vi "Item.vi"(8 "error in (no error)":errorcluster, 10 "Index":i32, 11 "ListImp in":refnum<class "ListImp.lvclass">) -> (0 "error out":errorcluster, 1 "Item":refnum<class>, 3 "ListImp out":refnum<class "ListImp.lvclass">)   [LabVIEW 2017, in "LapDog.Collections.v0.Lists.lvlib" / "ListImp.lvclass"]
uses:
  ListImp.lvclass
  ListImp.lvclass/ListImp.ctl
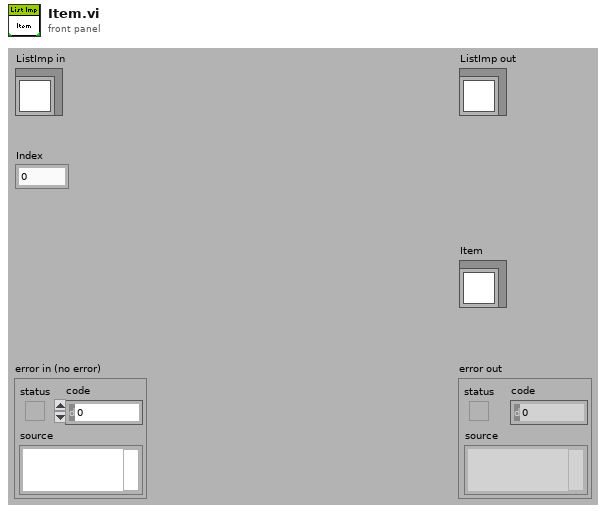
[diagram p1: front panel]
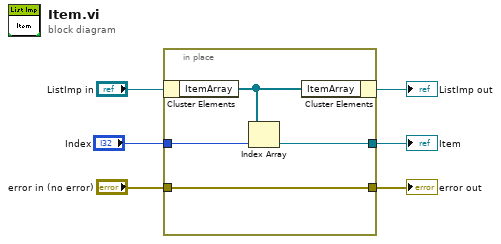
[diagram p0: block diagram]
diagram:
  n1 = in-place {
    in-place-border: [w10] -> w6
    in-place-border: "error in (no error)" -> [w9]
    in-place-border: [w9] -> w4
    in-place-border: "Index" -> [w8]
    n2 = in-place-cluster #1("ListImp in") -> ("ItemArray"=w7:refnum<class>[])
    n3 = Index Array(array=w7, index=w8) -> (element=w10:refnum<class>)
    n4 = in-place-cluster #1("ItemArray"=w7) -> (→"ListImp out":refnum<class "ListImp.lvclass">)
  }
  "error out" <- w4
  "Item" <- w6
